vi "Load Python Version and Path.vi"() -> (2 "path":path, 3 "version":string)   [LabVIEW 2025]
uses:
  <vilib>/Utility/config.llb/NI_LVConfig.lvlib
  <vilib>/Utility/config.llb/Read Key (String).vi
  <vilib>/Utility/config.llb/Read Key (Path).vi
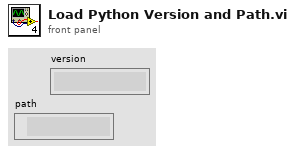
[diagram p1: front panel]
types:
  T1 = typedef "NI_LVConfig.lvlib/Config Data RefNum.ctl" = refnum<k1>
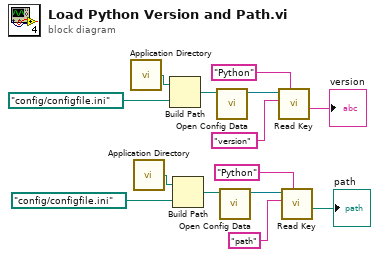
[diagram p0: block diagram]
diagram:
  n1 = call <vilib>:"Application Directory.vi"() -> ("Application Directory"=w14:path)
  n2 = call <vilib>:"Application Directory.vi"() -> ("Application Directory"=w7:path)
  n3 = Build Path(base path=w14, name or relative path=path "config/configfile.ini") -> (appended path=w12:path)
  n4 = Build Path(base path=w7, name or relative path=path "config/configfile.ini") -> (appended path=w5:path)
  n5 = call <vilib>:"Open Config Data.vi"("configuration file path"=w12) -> ("refnum"=w9:T1)  [unwired: 8 in, 2 out]
  n6 = call <vilib>:"Open Config Data.vi"("configuration file path"=w5) -> ("refnum"=w3:T1)  [unwired: 8 in, 2 out]
  n7 = call-poly <vilib>:"Read Key.vi"("section"="Python", "key"="version", "refnum"=w9) -> ("value"=→"version":string)  [unwired: 5 in, 3 out]
  n8 = call-poly <vilib>:"Read Key.vi"("section"="Python", "key"="path", "refnum"=w3) -> ("value"=→"path":path)  [unwired: 5 in, 3 out]
